vi "Create Properties Cluster.vi"(8 "error in":errorcluster, 11 "Node In":refnum<k20>) -> (0 "error out":errorcluster, 2 "Clust Refnum":refnum<vi>, 3 "Node Out":refnum<k20>)   [LabVIEW 2026, in "Plugin XML Parser.lvlib"]
uses:
  Plugin XML Parser.lvlib
  <vilib>/numeric/LVNumericRepresentation.ctl
  <vilib>/xml/Close Reference(Node).vi
  <resource>/objmgr/DOMUserDefRef.rc
  <vilib>/xml/NI_XML.lvlib
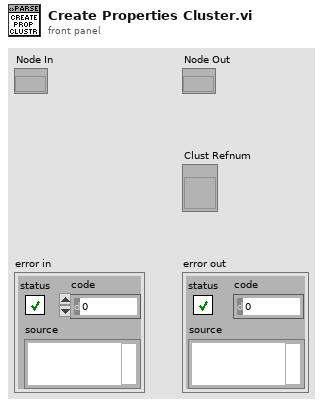
[diagram p1: front panel]
types:
  T1 = typedef "LVNumericRepresentation.ctl" = enum32{"Extended Precision", "Double Precision", "Single Precision", "Long", "Word", "Byte", "Unsigned Long", "Unsigned Word", "Unsigned Byte", "Complex Extended", "Complex Double", "Complex Single", "Quad", "Unsigned Quad", "Fixed-Point"}
  T2 = enum16{"String", "BinaryString", "Boolean", "I32", "I16", "I64", "U32", "U16", "Double", "U64", "Variant", "DependentNode", "DataSourceNode", "DependentFile", "BooleanArray", "U64Array", "U32Array", "U16Array", "DoubleArray", "I64Array", "I32Array", "I16Array", "StringArray", "Enum", "Dictionary", "DictionaryArray", "None"}
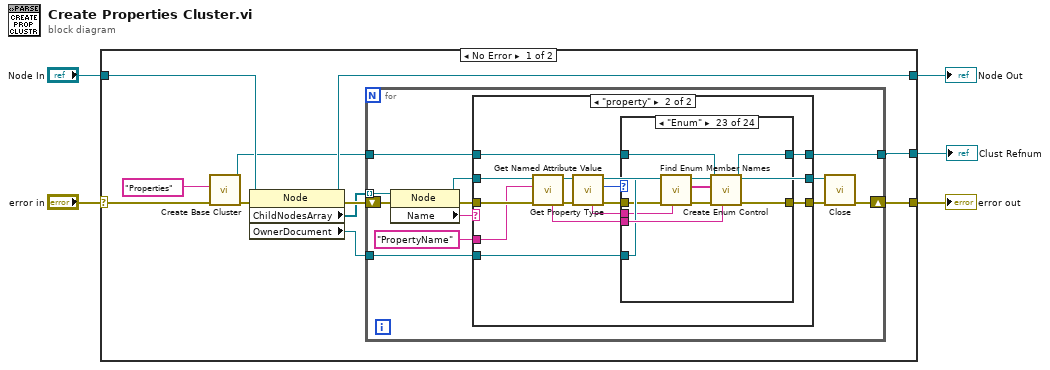
[diagram p0: block diagram]
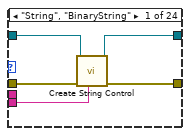
[diagram p3: hidden frame]
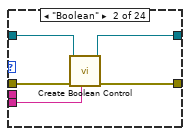
[diagram p4: hidden frame]
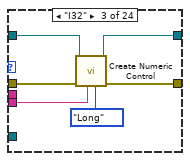
[diagram p5: hidden frame]
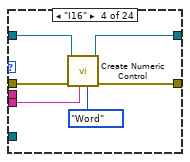
[diagram p6: hidden frame]
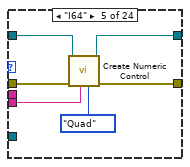
[diagram p7: hidden frame]
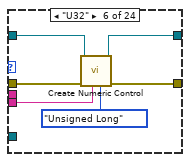
[diagram p8: hidden frame]
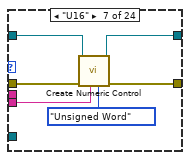
[diagram p9: hidden frame]
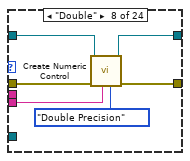
[diagram p10: hidden frame]
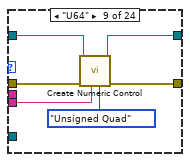
[diagram p11: hidden frame]
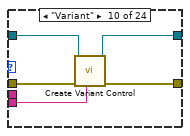
[diagram p12: hidden frame]
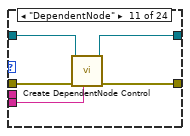
[diagram p13: hidden frame]
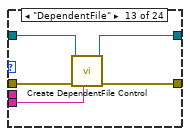
[diagram p15: hidden frame]
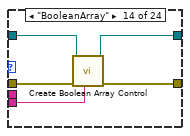
[diagram p16: hidden frame]
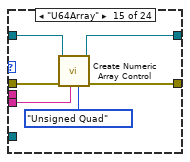
[diagram p17: hidden frame]
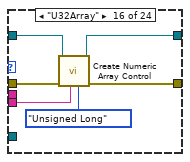
[diagram p18: hidden frame]
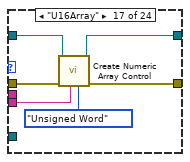
[diagram p19: hidden frame]
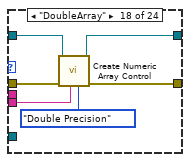
[diagram p20: hidden frame]
diagram:
  n1 = case shown="No Error" "error in" {
    selector: "error in" -> [w7 w179]
    tunnel: [w15 w179] -> w4
    tunnel: "Node In" -> [w14 w178]
    tunnel: [w13 w178] -> w2
    tunnel: [w11 _] -> w1
    frame No Error {
      n2 = call "Create Base Cluster.vi"("error in"=w7, "Cluster Name"="Properties") -> ("error out"=w8:errorcluster, "Cluster out"=w9:refnum<vi>)  [unwired: 7 in, 1 out]
      n3 = property class="Node"(reference=w14, error in=w8) -> (reference out=w13:refnum<k20>, error out=w16:errorcluster, "ChildNodesArray"=w12:refnum<k20>[], "OwnerDocument"=w6:refnum<k20>)
      n4 = for {
        tunnel: w9 -> [w20]
        shift-right: [w25] -> w15
        shift-left: w16 -> [w28]
        tunnel: w12 -> [w24] mode=indexing
        tunnel: [w19] -> w11
        tunnel: w6 -> [w17]
        n5 = property class="Node"(reference=w24, error in=w28) -> (reference out=w23:refnum<k20>, error out=w27:errorcluster, "Name"=w22:string)
        n6 = case shown="\"property\"" w22 {
          tunnel: w23 -> [w30 w39]
          tunnel: w27 -> [w31 w38]
          tunnel: [w31 w44] -> w26
          tunnel: [w30 w43] -> w21
          tunnel: w20 -> [w29 w42]
          tunnel: [w29 w40] -> w19
          tunnel: "PropertyName" ("Attribute Name") -> [_ w34]
          tunnel: w17 -> [_ w32]
          frame Default {
          }
          frame "property" {
            n7 = call "Get Named Attribute Value.vi"("error in"=w38, "Attribute Name"=w34, "Node In"=w39) -> ("error out"=w37:errorcluster, "Node Out"=w35:refnum<k20>, "Attribute Value"=w36:string)  [unwired: 5 in, 1 out]
            n8 = call "Get Property Type.vi"("error in"=w37, "Node in"=w35) -> ("error out"=w45:errorcluster, "Type"=w41:T2, "Node out"=w43:refnum<k20>, "Enum TypeName"=w33:string)  [unwired: 6 in]
            n9 = case shown="\"Enum\"" w41 {
              tunnel: w45 -> [w50 w55 w61 w67 w73 w79 w85 w90 w97 w102 w107 w109 w114 w119 w125 w131 w137 w143 w149 w155 w161 w166 w169 w177]
              tunnel: w36 -> [w48 w53 w58 w64 w70 w76 w82 w89 w94 w98 w103 _ w110 w115 w121 w127 w133 w139 w145 w151 w157 w163 w173 _]
              tunnel: w42 -> [w47 w52 w59 w65 w71 w77 w83 w87 w95 w100 w105 w108 w112 w117 w123 w129 w135 w141 w147 w153 w159 w164 w174 w176]
              tunnel: [w49 w54 w60 w66 w72 w78 w84 w91 w96 w101 w106 w109 w113 w118 w124 w130 w136 w142 w148 w154 w160 w165 w175 w177] -> w44
              tunnel: [w46 w51 w57 w63 w69 w75 w81 w88 w93 w99 w104 w108 w111 w116 w122 w128 w134 w140 w146 w152 w158 w162 w172 w176] -> w40
              tunnel: w33 -> [_ _ _ _ _ _ _ _ _ _ _ _ _ _ _ _ _ _ _ _ _ _ w167 _]
              tunnel: w32 -> [_ _ _ _ _ _ _ _ _ _ _ _ _ _ _ _ _ _ _ _ _ _ w171 _]
              frame "String", "BinaryString" {
                n10 = call "Create String Control.vi"("Label.Text"=w48, "error in"=w50, "Cluster in"=w47) -> ("error out"=w49:errorcluster, "Cluster out"=w46:refnum<vi>)  [unwired: 7 in]
              }
              frame "Boolean" {
                n11 = call "Create Boolean Control.vi"("Label.Text"=w53, "error in"=w55, "Cluster in"=w52) -> ("error out"=w54:errorcluster, "Cluster out"=w51:refnum<vi>)  [unwired: 7 in]
              }
              frame "I32" {
                n12 = call "Create Numeric Control.vi"("Representation"=LVNumericRepresentation."Long", "Label.Text"=w58, "error in"=w61, "Cluster in"=w59) -> ("error out"=w60:errorcluster, "Cluster out"=w57:refnum<vi>)  [unwired: 6 in]
              }
              frame "I16" {
                n13 = call "Create Numeric Control.vi"("Representation"=LVNumericRepresentation."Word", "Label.Text"=w64, "error in"=w67, "Cluster in"=w65) -> ("error out"=w66:errorcluster, "Cluster out"=w63:refnum<vi>)  [unwired: 6 in]
              }
              frame "I64" {
                n14 = call "Create Numeric Control.vi"("Representation"=LVNumericRepresentation."Quad", "Label.Text"=w70, "error in"=w73, "Cluster in"=w71) -> ("error out"=w72:errorcluster, "Cluster out"=w69:refnum<vi>)  [unwired: 6 in]
              }
              frame "U32" {
                n15 = call "Create Numeric Control.vi"("Representation"=LVNumericRepresentation."Unsigned Long", "Label.Text"=w76, "error in"=w79, "Cluster in"=w77) -> ("error out"=w78:errorcluster, "Cluster out"=w75:refnum<vi>)  [unwired: 6 in]
              }
              frame "U16" {
                n16 = call "Create Numeric Control.vi"("Representation"=LVNumericRepresentation."Unsigned Word", "Label.Text"=w82, "error in"=w85, "Cluster in"=w83) -> ("error out"=w84:errorcluster, "Cluster out"=w81:refnum<vi>)  [unwired: 6 in]
              }
              frame "Double" {
                n17 = call "Create Numeric Control.vi"("Representation"=LVNumericRepresentation."Double Precision", "Label.Text"=w89, "error in"=w90, "Cluster in"=w87) -> ("error out"=w91:errorcluster, "Cluster out"=w88:refnum<vi>)  [unwired: 6 in]
              }
              frame "U64" {
                n18 = call "Create Numeric Control.vi"("Representation"=LVNumericRepresentation."Unsigned Quad", "Label.Text"=w94, "error in"=w97, "Cluster in"=w95) -> ("error out"=w96:errorcluster, "Cluster out"=w93:refnum<vi>)  [unwired: 6 in]
              }
              frame "Variant" {
                n19 = call "Create Variant Control.vi"("Property Name"=w98, "error in"=w102, "Clust Refnum"=w100) -> ("error out"=w101:errorcluster, "Clust Refnum"=w99:refnum<vi>)  [unwired: 7 in]
              }
              frame "DependentNode" {
                n20 = call "Create DependentNode Control.vi"("Property Name"=w103, "error in"=w107, "Clust Refnum"=w105) -> ("error out"=w106:errorcluster, "Clust Refnum"=w104:refnum<vi>)  [unwired: 7 in]
              }
              frame "DataSourceNode" {
              }
              frame "DependentFile" {
                n21 = call "Create DependentFile Control.vi"("Property Name"=w110, "error in"=w114, "Clust Refnum"=w112) -> ("error out"=w113:errorcluster, "Clust Refnum"=w111:refnum<vi>)  [unwired: 7 in]
              }
              frame "BooleanArray" {
                n22 = call "Create Boolean Array Control.vi"("Property Name"=w115, "error in"=w119, "Clust Refnum"=w117) -> ("error out"=w118:errorcluster, "Clust Refnum"=w116:refnum<vi>)  [unwired: 7 in]
              }
              frame "U64Array" {
                n23 = call "Create Numeric Array Control.vi"("Representation"=LVNumericRepresentation."Unsigned Quad", "Property Name"=w121, "error in"=w125, "Clust Refnum"=w123) -> ("error out"=w124:errorcluster, "Clust Refnum"=w122:refnum<vi>)  [unwired: 6 in]
              }
              frame "U32Array" {
                n24 = call "Create Numeric Array Control.vi"("Representation"=LVNumericRepresentation."Unsigned Long", "Property Name"=w127, "error in"=w131, "Clust Refnum"=w129) -> ("error out"=w130:errorcluster, "Clust Refnum"=w128:refnum<vi>)  [unwired: 6 in]
              }
              frame "U16Array" {
                n25 = call "Create Numeric Array Control.vi"("Representation"=LVNumericRepresentation."Unsigned Word", "Property Name"=w133, "error in"=w137, "Clust Refnum"=w135) -> ("error out"=w136:errorcluster, "Clust Refnum"=w134:refnum<vi>)  [unwired: 6 in]
              }
              frame "DoubleArray" {
                n26 = call "Create Numeric Array Control.vi"("Representation"=LVNumericRepresentation."Double Precision", "Property Name"=w139, "error in"=w143, "Clust Refnum"=w141) -> ("error out"=w142:errorcluster, "Clust Refnum"=w140:refnum<vi>)  [unwired: 6 in]
              }
              frame "I64Array" {
                n27 = call "Create Numeric Array Control.vi"("Representation"=LVNumericRepresentation."Quad", "Property Name"=w145, "error in"=w149, "Clust Refnum"=w147) -> ("error out"=w148:errorcluster, "Clust Refnum"=w146:refnum<vi>)  [unwired: 6 in]
              }
              frame "I32Array" {
                n28 = call "Create Numeric Array Control.vi"("Representation"=LVNumericRepresentation."Long", "Property Name"=w151, "error in"=w155, "Clust Refnum"=w153) -> ("error out"=w154:errorcluster, "Clust Refnum"=w152:refnum<vi>)  [unwired: 6 in]
              }
              frame "I16Array" {
                n29 = call "Create Numeric Array Control.vi"("Representation"=LVNumericRepresentation."Word", "Property Name"=w157, "error in"=w161, "Clust Refnum"=w159) -> ("error out"=w160:errorcluster, "Clust Refnum"=w158:refnum<vi>)  [unwired: 6 in]
              }
              frame "StringArray" {
                n30 = call "Create String Array Control.vi"("Property Name"=w163, "error in"=w166, "Clust Refnum"=w164) -> ("error out"=w165:errorcluster, "Clust Refnum"=w162:refnum<vi>)  [unwired: 7 in]
              }
              frame "Enum" {
                n31 = call "Find Enum Member Names.vi"("Enum TypeName"=w167, "error in"=w169, "Doc Ref"=w171) -> ("error out"=w170:errorcluster, "EnumMembers"=w168:string[])  [unwired: 7 in]
                n32 = call "Create Enum Control.vi"("Property Name"=w173, "error in"=w170, "Enum Members"=w168, "Clust Refnum"=w174) -> ("error out"=w175:errorcluster, "Clust Refnum"=w172:refnum<vi>)  [unwired: 6 in]
              }
              frame "Dictionary".."None" {
              }
            }
          }
        }
        n33 = call-poly <vilib>:"Close.vi"("error in (no error)"=w26, "node"=w21) -> ("error out"=w25:errorcluster)  [unwired: 7 in]
      }
    }
    frame Error {
    }
  }
  "Node Out" <- w2
  "error out" <- w4
  "Clust Refnum" <- w1
